vi "Motion_Convert Double to Register.vi"(10 "Double Value":dbl format="%_7g") -> (2 "U16 Array":u16[](array[numeric]))   [LabVIEW 2010]
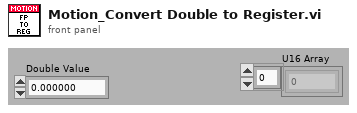
[diagram p1: front panel]
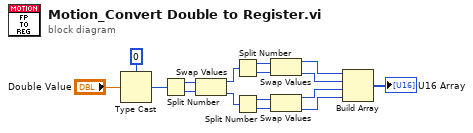
[diagram p0: block diagram]
diagram:
  n1 = Type Cast(type=i64 0, x="Double Value") -> (*(type *) &x=w14:i64)
  n2 = Split Number(x=w14) -> (hi(x)=w4:u32, lo(x)=w2:u32)
  n3 = Swap Values(12:w4, 14:w2) -> (1:w1:u32, 3:w3:u32)  [unwired: 1 in]
  n4 = Split Number(x=w1) -> (hi(x)=w12:u16, lo(x)=w10:u16)
  n5 = Split Number(x=w3) -> (hi(x)=w8:u16, lo(x)=w6:u16)
  n6 = Swap Values(12:w12, 14:w10) -> (1:w9:u16, 3:w11:u16)  [unwired: 1 in]
  n7 = Swap Values(12:w8, 14:w6) -> (1:w5:u16, 3:w7:u16)  [unwired: 1 in]
  n8 = Build Array(w9, w11, w5, w7) -> (→"U16 Array":u16[])
